vi "ProducerConsumerExample.vi"() -> ()   [LabVIEW 2010]
doc: "Use this template to build a producer/consumer design pattern. Use this template when you need to execute a process, such as data analysis, when a data source, such as a triggered acquisition, produces data at an uneven rate and you need to execute the process when the data becomes available."
uses:
  <vilib>/DAQmx/write.llb/DAQmx Write (Analog 1D DBL 1Chan NSamp).vi
  <vilib>/DAQmx/read.llb/DAQmx Read (Counter 1D U32 1Chan NSamp).vi
  <vilib>/DAQmx/create/channels.llb/DAQmx Create Channel (CI-Count Edges).vi
  <vilib>/DAQmx/create/channels.llb/DAQmx Create Channel (AO-Voltage-Basic).vi
  <vilib>/DAQmx/configure/timing.llb/DAQmx Timing (Sample Clock).vi
  <vilib>/daqmx/miscellaneous.llb/DAQmx Fill In Error Info.vi
panel:
  out "Waveform Chart":u32[](graph)
  in  "stop":bool
  # "X-Axis has been autoscaled"
  # "This example has been written to acquire data from a 100 Hz Sine Wave.\nYou can use a Test Panel in the  Measurement and Automation Explorer\nto generate a 100 Hz Sine Wave; however, you will need to connect\nthe AO channel where the waveform is generated with the AI channel\nthat you want to use to read the waveform data into LabVIEW."
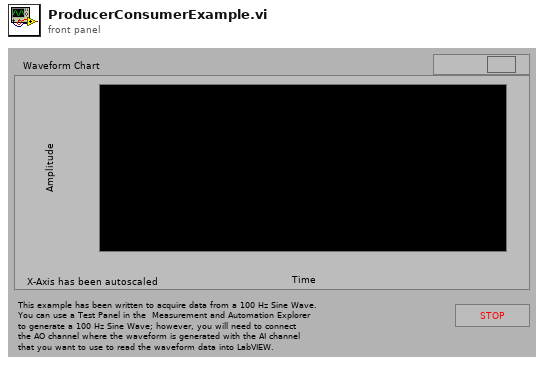
[diagram p1: front panel]
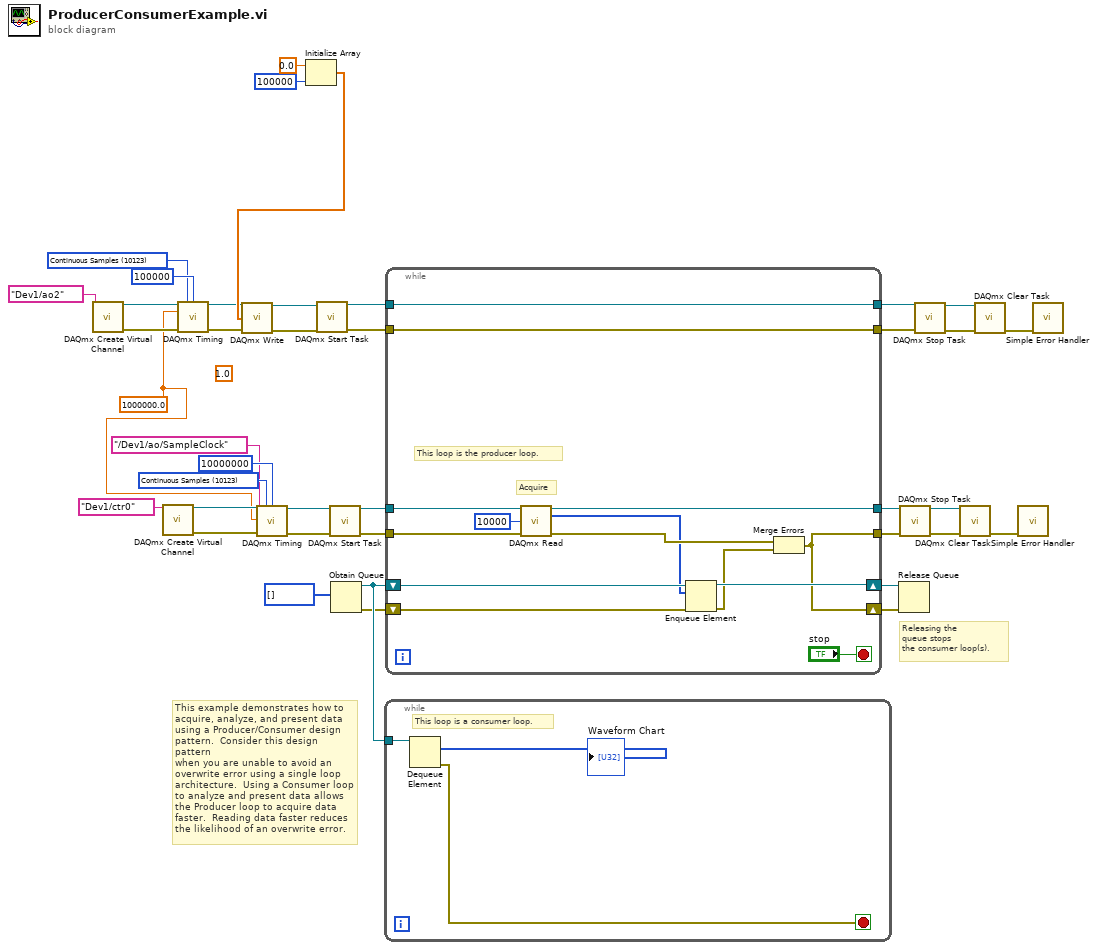
[diagram p0: block diagram]
diagram:
  (unwired) 1.0 ("data")
  w17 = 10123 items=["Finite Samples"=10178, "Continuous Samples"=10123, "Hardware Timed Single Point"=12522] ("sample mode")
  w1 = 1000000.0 ("rate")
  w30 = 10123 items=["Finite Samples"=10178, "Continuous Samples"=10123, "Hardware Timed Single Point"=12522] ("sample mode")
  # "This example demonstrates how to\nacquire, analyze, and present data\nusing a Producer/Consumer design\npattern.  Consider this design pattern\nwhen you are unable to avoid an \noverwrite error using a single loop\narchitecture.  Using a Consumer loop\nto analyze and present data allows\nthe Producer loop to acquire data\nfaster.  Reading data faster reduces\nthe likelihood of an overwrite error."
  # "Releasing the\nqueue stops\nthe consumer loop(s)."
  n1 = call-poly <vilib>:"DAQmx Create Virtual Channel.vi"("physical channels"=tag "Dev1/ao2") -> ("task out"=w19:refnum<k21>, "error out"=w11:errorcluster)  [unwired: 13 in]
  n2 = call-poly <vilib>:"DAQmx Create Virtual Channel.vi"("counter"=tag "Dev1/ctr0") -> ("task out"=w34:refnum<k21>, "error out"=w33:errorcluster)  [unwired: 13 in]
  n3 = call-poly <vilib>:"DAQmx Timing.vi"("task/channels in"=w19, "sample mode"=w17, "samples per channel"=100000, "rate"=w1, "error in"=w11) -> ("task out"=w13:refnum<k21>, "error out"=w12:errorcluster)  [unwired: 9 in]
  n4 = call-poly <vilib>:"DAQmx Timing.vi"("task/channels in"=w34, "sample mode"=w30, "samples per channel"=10000000, "rate"=w1, "source"=tag "/Dev1/ao/SampleClock", "error in"=w33) -> ("task out"=w32:refnum<k21>, "error out"=w31:errorcluster)  [unwired: 8 in]
  n5 = Initialize Array(0.0 ("element"), 100000 ("dimension size")) -> (w14:dbl[])
  n6 = call-poly <vilib>:"DAQmx Write.vi"("task/channels in"=w13, "data"=w14, "error in"=w12) -> ("task out"=w10:refnum<k21>, "error out"=w9:errorcluster)  [unwired: 10 in, 1 out]
  n7 = call <vilib>:"DAQmx Start Task.vi"("task/channels in"=w10, "error in"=w9) -> ("task out"=w8:refnum<k21>, "error out"=w7:errorcluster)  [unwired: 12 in]
  n8 = call <vilib>:"DAQmx Start Task.vi"("task/channels in"=w32, "error in"=w31) -> ("task out"=w29:refnum<k21>, "error out"=w28:errorcluster)  [unwired: 12 in]
  n9 = Obtain Queue(element data type=u32[] [] ("Array")) -> (queue out=w40:refnum<queue>, error out=w39:errorcluster)  [unwired: 4 in, 1 out]
  n10 = while {
    tunnel: w40 -> [w43]
    stop <- w42 stop-if-true
    # "This loop is a consumer loop."
    n11 = Dequeue Element(queue=w43) -> (element=→"Waveform Chart":u32[], error out=w42:errorcluster)  [unwired: 2 in, 2 out]
  }
  n12 = while {
    shift-right: [w47] -> w37
    shift-left: w39 -> [w54]
    shift-right: [w55] -> w38
    shift-left: w40 -> [w56]
    tunnel: w29 -> [w53]
    tunnel: w28 -> [w52]
    tunnel: [w48] -> w26
    tunnel: [w47] -> w25
    tunnel: [w45] -> w3
    tunnel: w8 -> [w45]
    tunnel: w7 -> [w44]
    tunnel: [w44] -> w2
    stop <- "stop" stop-if-true
    # "Acquire"
    # "This loop is the producer loop."
    n13 = call-poly <vilib>:"DAQmx Read.vi"("task/channels in"=w53, "number of samples per channel"=10000, "error in"=w52) -> ("task out"=w48:refnum<k21>, "data"=w49:u32[], "error out"=w51:errorcluster)  [unwired: 10 in]
    n14 = Enqueue Element(queue=w56, element=w49, error in (no error)=w54) -> (queue out=w55:refnum<queue>, error out=w50:errorcluster)  [unwired: 1 in, 1 out]
    n15 = Merge Errors(w51, w50) -> (w47:errorcluster)
  }
  n16 = Release Queue(queue=w38, error in (no error)=w37) -> ()  [unwired: 1 in, 3 out]
  n17 = call <vilib>:"DAQmx Stop Task.vi"("task/channels in"=w26, "error in"=w25) -> ("task out"=w35:refnum<k21>, "error out"=w36:errorcluster)  [unwired: 12 in]
  n18 = call <vilib>:"DAQmx Stop Task.vi"("task/channels in"=w3, "error in"=w2) -> ("task out"=w5:refnum<k21>, "error out"=w4:errorcluster)  [unwired: 12 in]
  n19 = call <vilib>:"DAQmx Clear Task.vi"("task in"=w35, "error in"=w36) -> ("error out"=w24:errorcluster)  [unwired: 13 in]
  n20 = call <vilib>:"DAQmx Clear Task.vi"("task in"=w5, "error in"=w4) -> ("error out"=w6:errorcluster)  [unwired: 13 in]
  n21 = call <vilib>:"Simple Error Handler.vi"("error in (no error)"=w24) -> ()  [unwired: 4 in, 5 out]
  n22 = call <vilib>:"Simple Error Handler.vi"("error in (no error)"=w6) -> ()  [unwired: 4 in, 5 out]
